vi "Load_File.vi"() -> ()   [LabVIEW 2020, in "Chip_Analyze.lvlib"]
uses:
  Chip_Analyze.lvlib
  <vilib>/Utility/file.llb/Read Delimited Spreadsheet (DBL).vi
panel:
  out "Result":string[][](array[string])
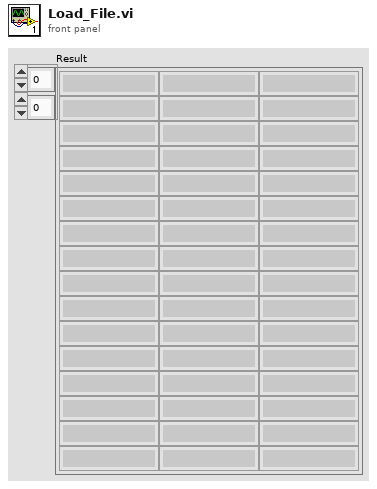
[diagram p1: front panel]
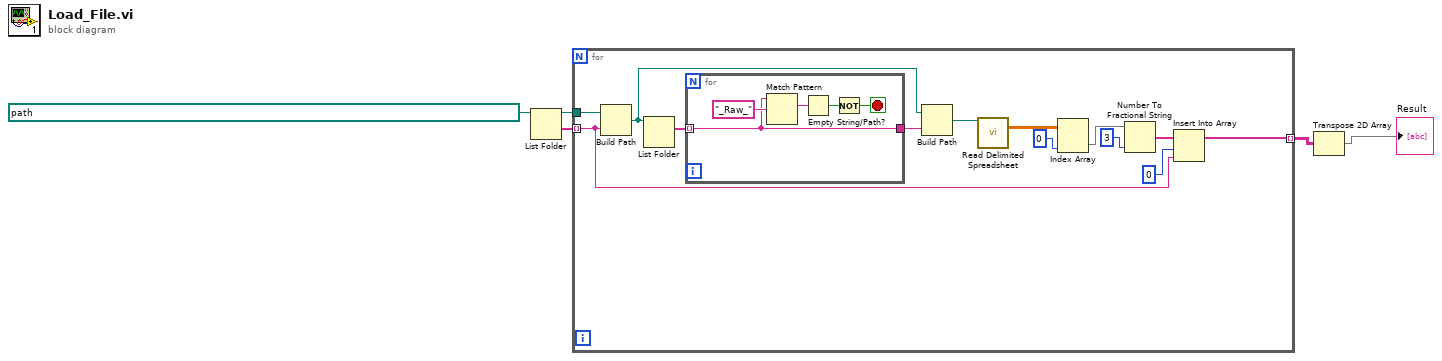
[diagram p0: block diagram]
diagram:
  n1 = List Folder(path=path "C:/Users/georg/Desktop/光核心/2022.05.27 New Hg-Ar Auto Program/0527/DATA/0628") -> (path out=w4:path, folder names=w3:string[])  [unwired: 3 in, 2 out]
  n2 = for {
    tunnel: w3 -> [w8] mode=indexing
    tunnel: w4 -> [w18]
    tunnel: [w6] -> w2 mode=indexing
    n3 = Build Path(base path=w18, name or relative path=w8) -> (appended path=w16:path)
    n4 = List Folder(path=w16) -> (filenames=w17:string[])  [unwired: 3 in, 3 out]
    n5 = for {
      tunnel: w17 -> [w21] mode=indexing
      tunnel: [w21] -> w15
      stop <- w19 stop-if-true
      n6 = Match Pattern(string=w21, regular expression="_Raw_") -> (match substring=w22:string)  [unwired: 1 in, 3 out]
      n7 = Empty String/Path?(string/path=w22) -> (empty?=w20:bool)
      n8 = Not(x=w20) -> (.not. x?=w19:bool)
    }
    n9 = Build Path(base path=w16, name or relative path=w15) -> (appended path=w14:path)
    n10 = call-poly <vilib>:"Read Delimited Spreadsheet.vi"("file path (dialog if empty)"=w14) -> ("all rows"=w13:dbl[][])  [unwired: 9 in, 5 out]
    n11 = Index Array(array=w13, index (col)=0 ("disabled index (col)")) -> (element=w11:dbl[])  [unwired: 1 in]
    n12 = Number To Fractional String(number=w11, precision (6)=i16 3) -> (F-format string=w10:string[])  [unwired: 2 in]
    n13 = Insert Into Array(array=w10, index=0, new element=w8) -> (w6:string[])
  }
  n14 = Transpose 2D Array(2D array=w2) -> (transposed array=→"Result":string[][])
